vi "ColorSensor Controller.vi"(8 "error in":errorcluster) -> ()   [LabVIEW 2019]
doc: "This VI executes continuously carrying out the current operation and responding to updates or new operations. It will often contain the timing or control code that is difficult to place directly in TeleOp. This VI generally opens all sensors and motors and isolates the rest of the robot code from knowing how the operations are carried out."
uses:
  <vilib>/Rock Robotics/WPI/Framework/Completion Status.ctl
  ColorSensor Setpoints.ctl
  ColorSensor Operations.ctl
  <vilib>/Rock Robotics/SystemInterfaces/i2clib/i2c_bus.ctl
  <vilib>/Rock Robotics/WPI/ThirdParty/Phoenix-LabVIEW/Motor Controller/Controls/CTRE_Phoenix_MotorControl_ControlMode.ctl
  Framework/Robot Global Data.vi
  <vilib>/Rock Robotics/Network Tables/NT Write Boolean.vi
panel:
  in  "Interactive Values":T1
  out "Current\nCmd":string
  in  "Buttons":cluster{"Execute Cmd":bool, "Abort Cmd":bool}
  out "Command Timing":cluster{"Start Time (ms)":u32, "Iterations":i32}
  out "Status":T3
  # "Tip: It may be helpful to observe inputs and sensor values.\nYou may also want to display tuning or debugging controls."
  # "Interactive Command: You may fill in the settings for a command\nand schedule it with the Execute button. You can observe and abort\nany command while fine tuning the code for the controller."
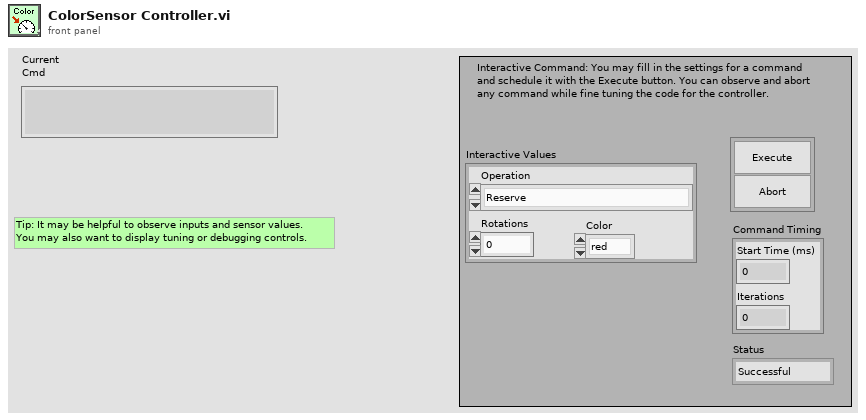
[diagram p1: front panel]
types:
  T1 = typedef "ColorSensor Setpoints.ctl" = cluster{"Operation":T2, "Rotations":dbl, "Color":enum16{"red", "blue", "yellow", "green"}}
  T2 = typedef "ColorSensor Operations.ctl" = enum16{"Reserve", "Read Current", "spin_to_color", "ColorSpin", "Immediate"}
  T3 = typedef "Completion Status.ctl" = enum16{"Successful", "Aborted", "Incomplete"}
  T4 = typedef "i2c_bus.ctl" = enum16{"I2C On-Board", "I2C MXP", "Invalid"}
  T5 = typedef "Color Sensor V3 DevRef.ctl" = cluster{"I2CDevRef":T6}
  T6 = typedef "WPI_I2CDevRef.ctl" = cluster{"DevStatus":errorcluster, "Device Address":u8, "Handle":i32, "I2C Bus":T4}
  T7 = typedef "WPI_MotorControlDeviceRef.ctl" = cluster{"DeviceStatus":errorcluster, "Type":T8, "PWM":cluster{"PWM Channel":T9, "DeadBand":T10}, "CAN":cluster{"Device Number":u8, "SetOutput VI Ref":variant, "GetOutput VI Ref":variant, "Enable VI Ref":variant, "Disable VI Ref":variant, "Data":variant}, "Invert":bool, "DIO PWM":cluster{"PWM \"Enable\" Channel":T9, "DIOChannel":T11, "PWM Rate":dbl}}
  T8 = typedef "WPI_MotorControlType.ctl" = enum16{"PWM", "CAN", "DIO PWM"}
  T9 = typedef "FPGA_DIOPWMChannel.ctl" = enum8{"PWM 0", "PWM 1", "PWM 2", "PWM 3", "PWM 4", "PWM 5", "PWM 6", "PWM 7", "PWM 8", "PWM 9", "PWM MXP 0", "PWM MXP 1", "PWM MXP 2", "PWM MXP 3", "PWM MXP 4", "PWM MXP 5", "PWM MXP 6", "PWM MXP 7", "PWM MXP 8", "PWM MXP 9", "Invalid"}
  T10 = typedef "WPI_PWMDeadband.ctl" = cluster{"Name":string, "maxPositivePwm":i32, "minPositivePwm":i32, "centerPwm":i32, "maxNegativePwm":i32, "minNegativePwm":i32, "angularRange":u16}
  T11 = typedef "FPGA_DIOChannel.ctl" = enum8{"DIO 0", "DIO 1", "DIO 2", "DIO 3", "DIO 4", "DIO 5", "DIO 6", "DIO 7", "DIO 8", "DIO 9", "DIO MXP 0", "DIO MXP 1", "DIO MXP 2", "DIO MXP 3", "DIO MXP 4", "DIO MXP 5", "DIO MXP 6", "DIO MXP 7", "DIO MXP 8", "DIO MXP 9", "DIO MXP 10", "DIO MXP 11", "DIO MXP 12", "DIO MXP 13", "DIO MXP 14", "DIO MXP 15", "SPI Port CS1", "SPI Port CS2", "SPI Port CS3", "SPI Port MISO", "SPI Port MOSI", "Invalid"}
  T12 = typedef "Command Status Info.ctl" = cluster{"Name":string, "Status":T3, "notifier out":T13}
  T13 = typedef "Completion Notifier.ctl" = refnum<notifier>
  T14 = cluster{"Current Command":T1, "Command Timing":cluster{"Start Time (ms)":u32, "Iterations":i32}, "Command Arguments":cluster{"Command Info":T12, "Description":string, "Default Command":T1, "queue out":refnum<queue>, "Subsystem Name":string}}
  T15 = typedef "CTRE_Phoenix_MotorControl_ControlMode.ctl" = u16
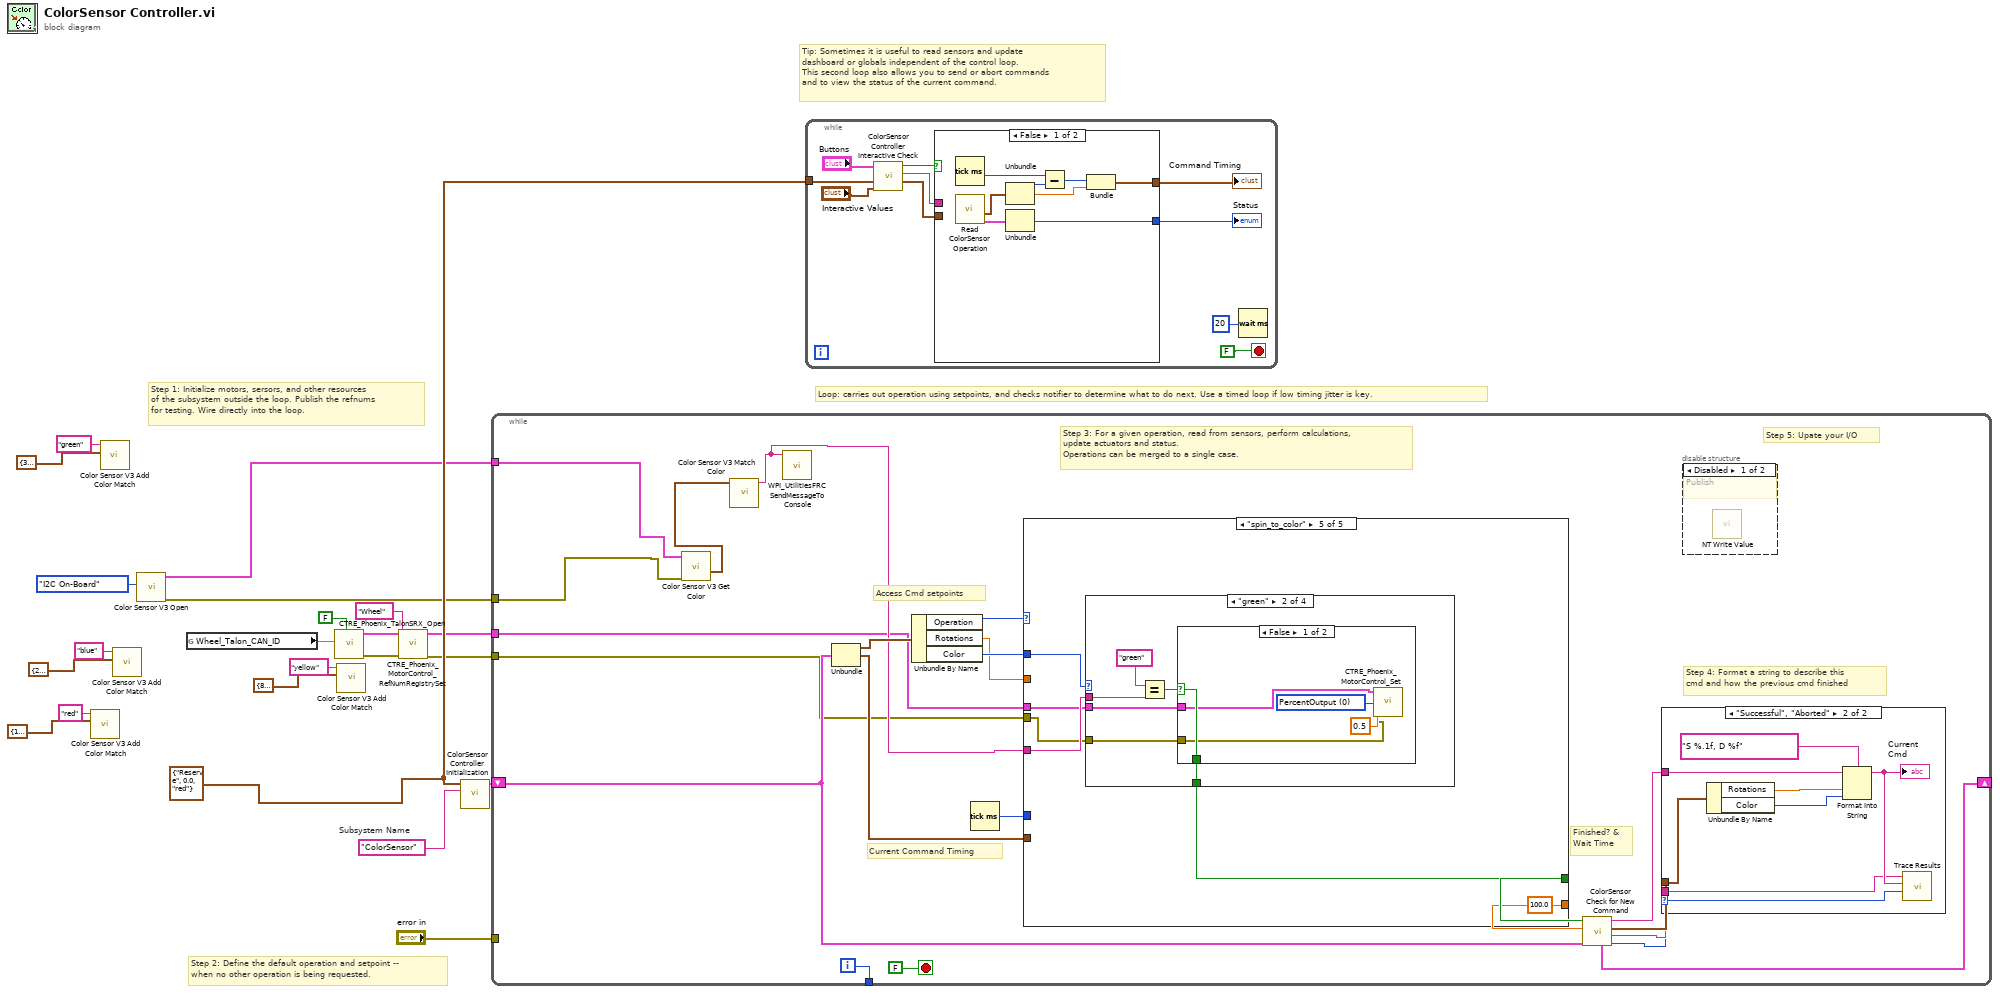
[diagram p0: block diagram]
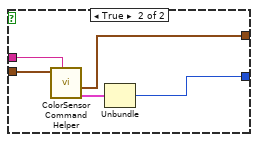
[diagram p2: hidden frame]
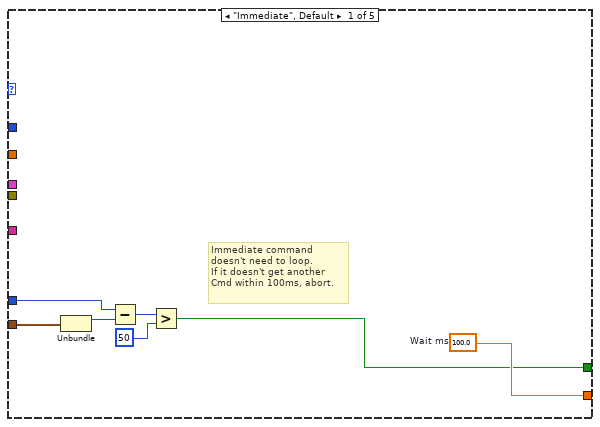
[diagram p5: hidden frame]
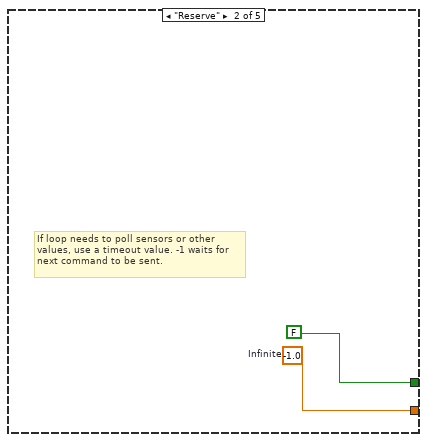
[diagram p6: hidden frame]
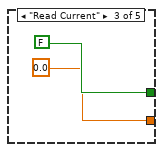
[diagram p7: hidden frame]
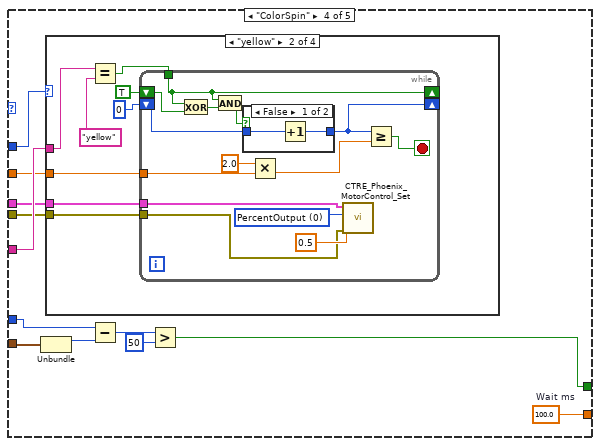
[diagram p8: hidden frame]
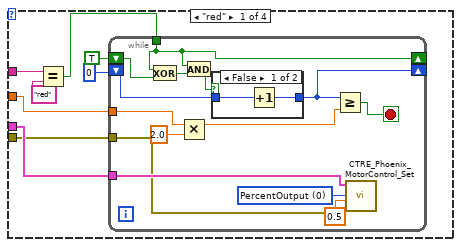
[diagram p9: hidden frame]
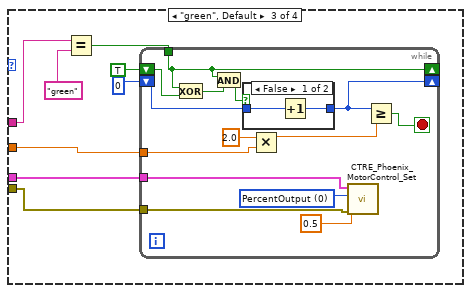
[diagram p12: hidden frame]
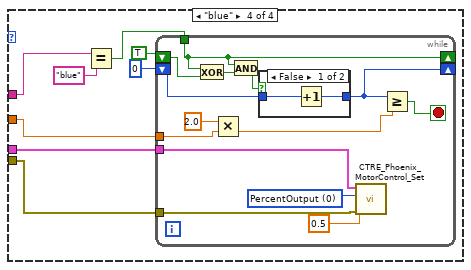
[diagram p14: hidden frame]
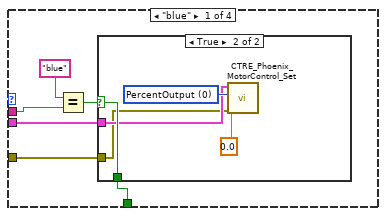
[diagram p16: hidden frame]
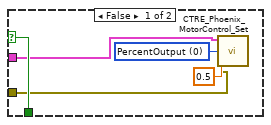
[diagram p17: hidden frame]
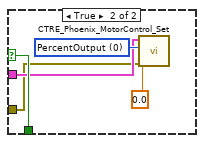
[diagram p18: hidden frame]
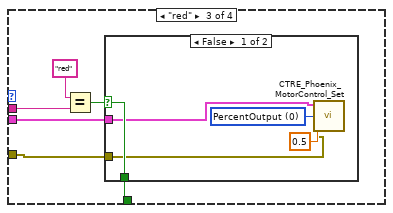
[diagram p19: hidden frame]
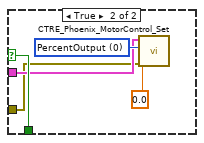
[diagram p20: hidden frame]
diagram:
  w16 = T1 {"Operation"=enum."Reserve", "Rotations"=0.0, "Color"=enum."red"} ("Default Command")
  w20 = "ColorSensor"  # Subsystem Name
  # "Tip: Sometimes it is useful to read sensors and update\ndashboard or globals independent of the control loop.\nThis second loop also allows you to send or abort commands\nand to view the status of the current command."
  # "Step 2: Define the default operation and setpoint --\nwhen no other operation is being requested."
  # "Step 1: Initialize motors, sersors, and other resources\nof the subsystem outside the loop. Publish the refnums\nfor testing. Wire directly into the loop."
  # "Loop: carries out operation using setpoints, and checks notifier to determine what to do next. Use a timed loop if low timing jitter is key."
  n1 = call <vilib>:"Color Sensor V3 Add Color Match.vi"("Color"=cluster{"R":dbl, "G":dbl, "B":dbl} {"R"=149.0, "G"=77.0, "B"=28.0}, "Name"="red") -> ()  [unwired: 10 in]
  n2 = call <vilib>:"Color Sensor V3 Add Color Match.vi"("Color"=cluster{"R":dbl, "G":dbl, "B":dbl} {"R"=39.0, "G"=149.0, "B"=66.0}, "Name"="green") -> ()  [unwired: 10 in]
  n3 = call <vilib>:"Color Sensor V3 Add Color Match.vi"("Color"=cluster{"R":dbl, "G":dbl, "B":dbl} {"R"=28.0, "G"=105.0, "B"=121.0}, "Name"="blue") -> ()  [unwired: 10 in]
  n4 = call <vilib>:"Color Sensor V3 Open.vi"("I2C Bus"=i2c_bus."I2C On-Board") -> ("error out"=w13:errorcluster, "ColorSensorDevRef"=w14:T5)  [unwired: 9 in]
  n5 = global read "Robot Global Data.vi" "Wheel_Talon_CAN_ID"() -> (w4:dbl)
  n6 = call <vilib>:"CTRE_Phoenix_TalonSRX_Open.vi"("Invert"=FALSE, "Device Number"=w4) -> ("error out"=w18:errorcluster, "CAN Talon SRX Ref"=w19:T7)  [unwired: 8 in]
  n7 = call <vilib>:"Color Sensor V3 Add Color Match.vi"("Color"=cluster{"R":dbl, "G":dbl, "B":dbl} {"R"=85.0, "G"=141.0, "B"=28.0}, "Name"="yellow") -> ()  [unwired: 10 in]
  n8 = call <vilib>:"CTRE_Phoenix_MotorControl_RefNumRegistrySet.vi"("error in (no error)"=w18, "refnum name"="Wheel", "PhoenixMotorControlDevRef"=w19) -> ("error out"=w1:errorcluster, "PhoenixMotorControlDevRef"=w2:T7)  [unwired: 7 in]
  n9 = call "ColorSensor Controller Initialization.vi"("Subsystem Name"=w20, "Default Command"=w16) -> ("Current Command"=w21:T14)  [unwired: 9 in]
  n10 = while {
    shift-right: [w38] -> _
    shift-left: w21 -> [w31]
    tunnel: [w43] -> _
    tunnel: "error in" -> [_]
    tunnel: w14 -> [w27]
    tunnel: w13 -> [w26]
    tunnel: w2 -> [w24]
    tunnel: w1 -> [w23]
    i -> [w43]
    stop <- FALSE stop-if-true
    # "Step 5: Upate your I/O"
    # "Step 4: Format a string to describe this\ncmd and how the previous cmd finished"
    # "Current Command Timing"
    # "Access Cmd setpoints"
    # "Finished? &\nWait Time"
    # "Step 3: For a given operation, read from sensors, perform calculations,\nupdate actuators and status.\nOperations can be merged to a single case."
    n11 = call <vilib>:"Color Sensor V3 Get Color.vi"("error in (no error)"=w26, "ColorSensorDevRef"=w27) -> ("Normalized Color"=w25:cluster{"R":dbl, "G":dbl, "B":dbl})  [unwired: 6 in, 3 out]
    n12 = call <vilib>:"Color Sensor V3 Match Color.vi"("Measured Color"=w25) -> ("Matched Color Name"=w28:string)  [unwired: 8 in, 2 out]
    n13 = call <vilib>:"WPI_UtilitiesFRC SendMessageToConsole.vi"("Message"=w28) -> ()  [unwired: 14 in, 1 out]
    n14 = Unbundle(w31) -> ("Current Command"=w42:T1, "Command Timing"=w39:cluster{"Start Time (ms)":u32, "Iterations":i32})  [unwired: 1 out]
    n15 = Unbundle By Name(w42) -> ("Operation"=w41:T2, "Rotations"=w29:dbl, "Color"=w30:enum16{"red", "blue", "yellow", "green"})
    n16 = Tick Count (ms)() -> (millisecond timer value=w40:u32)
    n17 = case shown="\"spin_to_color\"" w41 {
      tunnel: [w59 w61 0.0 ("Infinite") w68 100.0 ("Wait ms")] -> w36
      tunnel: [w53 FALSE ("ignore previous (F)") FALSE ("ignore previous (F)") w69 w180] -> w37
      tunnel: w39 -> [w55 _ _ w71 _]
      tunnel: w40 -> [w54 _ _ w70 _]
      tunnel: w28 -> [_ _ _ w73 w181]
      tunnel: w30 -> [_ _ _ w67 w178]
      tunnel: w29 -> [_ _ _ w66 _]
      tunnel: w24 -> [_ _ _ w65 w177]
      tunnel: w23 -> [_ _ _ w64 w176]
      frame "Immediate", Default {
        w59 = 100.0  # Wait ms
        # "Immediate command\ndoesn't need to loop.\nIf it doesn't get another\nCmd within 100ms, abort."
        n18 = Unbundle(w55) -> ("Start Time (ms)"=w58:u32)  [unwired: 1 out]
        n19 = Subtract(x=w54, y=w58) -> (x-y=w57:u32)
        n20 = Greater?(x=w57, y=u8 50 ("Left Motor")) -> (0:w53:bool)
      }
      frame "Reserve" {
        w61 = -1.0  # Infinite
        # "If loop needs to poll sensors or other\nvalues, use a timeout value. -1 waits for\nnext command to be sent."
      }
      frame "Read Current" {
      }
      frame "ColorSpin" {
        w68 = 100.0  # Wait ms
        n21 = Unbundle(w71) -> ("Start Time (ms)"=w72:u32)  [unwired: 1 out]
        n22 = case shown="\"yellow\"" w67 {
          tunnel: w73 -> [w79 w104 w129 w154]
          tunnel: w66 -> [w78 w103 w128 w153]
          tunnel: w65 -> [w77 w102 w127 w152]
          tunnel: w64 -> [w76 w101 w126 w151]
          frame "red" {
            n23 = Equal?(x=w79, y="red") -> (x = y?=w81:bool)
            n24 = while {
              shift-right: [w89] -> _
              shift-left: TRUE -> [w96]
              shift-right: [w93] -> _
              shift-left: 0 -> [w97]
              tunnel: w81 -> [w89]
              tunnel: w78 -> [w86]
              tunnel: w77 -> [w85]
              tunnel: w76 -> [w84]
              stop <- w92 stop-if-true
              w90 = T15 0 items=["PercentOutput"=0, "Position"=1, "Velocity"=2, "Current"=3, "Follower"=5, "MotionProfile"=6, "MotionMagic"=7, "MotionProfileArc"=10, "Disabled"=15] ("Control Mode")
              n25 = Exclusive Or(1:w96, 2:w89) -> (0:w95:bool)
              n26 = Multiply(x=w86, y=2.0) -> (x*y=w88:dbl)
              n27 = And(x=w89, y=w95) -> (x .and. y?=w94:bool)
              n28 = case shown="False" w94 {
                tunnel: w97 -> [w98 w100]
                tunnel: [w99 w100] -> w93
                frame False {
                  n29 = Increment(x=w98) -> (x+1=w99:i32)
                }
                frame True {
                }
              }
              n30 = Greater Or Equal?(x=w93, y=w88) -> (x >= y?=w92:bool)
              n31 = call <vilib>:"CTRE_Phoenix_MotorControl_Set.vi"("error in (no error)"=w84, "Output"=0.5, "Control Mode"=w90, "PhoenixMotorControlDevRef"=w85) -> ()  [unwired: 6 in, 2 out]
            }
          }
          frame "yellow" {
            n32 = Equal?(x=w104, y="yellow") -> (x = y?=w107:bool)
            n33 = while {
              shift-right: [w119] -> _
              shift-left: TRUE -> [w121]
              tunnel: w107 -> [w119]
              shift-right: [w117] -> _
              shift-left: 0 -> [w122]
              tunnel: w103 -> [w111]
              tunnel: w102 -> [w110]
              tunnel: w101 -> [w109]
              stop <- w116 stop-if-true
              w115 = T15 0 items=["PercentOutput"=0, "Position"=1, "Velocity"=2, "Current"=3, "Follower"=5, "MotionProfile"=6, "MotionMagic"=7, "MotionProfileArc"=10, "Disabled"=15] ("Control Mode")
              n34 = Exclusive Or(1:w121, 2:w119) -> (0:w120:bool)
              n35 = And(x=w119, y=w120) -> (x .and. y?=w118:bool)
              n36 = case shown="False" w118 {
                tunnel: w122 -> [w123 w125]
                tunnel: [w124 w125] -> w117
                frame False {
                  n37 = Increment(x=w123) -> (x+1=w124:i32)
                }
                frame True {
                }
              }
              n38 = Multiply(x=2.0, y=w111) -> (x*y=w113:dbl)
              n39 = call <vilib>:"CTRE_Phoenix_MotorControl_Set.vi"("error in (no error)"=w109, "Output"=0.5, "Control Mode"=w115, "PhoenixMotorControlDevRef"=w110) -> ()  [unwired: 6 in, 2 out]
              n40 = Greater Or Equal?(x=w117, y=w113) -> (x >= y?=w116:bool)
            }
          }
          frame "green", Default {
            n41 = Equal?(x=w129, y="green") -> (x = y?=w131:bool)
            n42 = while {
              shift-right: [w144] -> _
              shift-left: TRUE -> [w146]
              tunnel: w131 -> [w144]
              shift-right: [w142] -> _
              shift-left: 0 -> [w147]
              tunnel: w128 -> [w136]
              tunnel: w127 -> [w135]
              tunnel: w126 -> [w134]
              stop <- w141 stop-if-true
              w140 = T15 0 items=["PercentOutput"=0, "Position"=1, "Velocity"=2, "Current"=3, "Follower"=5, "MotionProfile"=6, "MotionMagic"=7, "MotionProfileArc"=10, "Disabled"=15] ("Control Mode")
              n43 = Exclusive Or(1:w146, 2:w144) -> (0:w145:bool)
              n44 = And(x=w144, y=w145) -> (x .and. y?=w143:bool)
              n45 = case shown="False" w143 {
                tunnel: w147 -> [w148 w150]
                tunnel: [w149 w150] -> w142
                frame False {
                  n46 = Increment(x=w148) -> (x+1=w149:i32)
                }
                frame True {
                }
              }
              n47 = Multiply(x=2.0, y=w136) -> (x*y=w138:dbl)
              n48 = call <vilib>:"CTRE_Phoenix_MotorControl_Set.vi"("error in (no error)"=w134, "Output"=0.5, "Control Mode"=w140, "PhoenixMotorControlDevRef"=w135) -> ()  [unwired: 6 in, 2 out]
              n49 = Greater Or Equal?(x=w142, y=w138) -> (x >= y?=w141:bool)
            }
          }
          frame "blue" {
            n50 = Equal?(x=w154, y="blue") -> (x = y?=w157:bool)
            n51 = while {
              shift-right: [w169] -> _
              shift-left: TRUE -> [w171]
              tunnel: w157 -> [w169]
              shift-right: [w167] -> _
              shift-left: 0 -> [w172]
              tunnel: w153 -> [w162]
              tunnel: w152 -> [w160]
              tunnel: w151 -> [w159]
              stop <- w166 stop-if-true
              w165 = T15 0 items=["PercentOutput"=0, "Position"=1, "Velocity"=2, "Current"=3, "Follower"=5, "MotionProfile"=6, "MotionMagic"=7, "MotionProfileArc"=10, "Disabled"=15] ("Control Mode")
              n52 = Exclusive Or(1:w171, 2:w169) -> (0:w170:bool)
              n53 = Multiply(x=2.0, y=w162) -> (x*y=w161:dbl)
              n54 = And(x=w169, y=w170) -> (x .and. y?=w168:bool)
              n55 = case shown="False" w168 {
                tunnel: w172 -> [w173 w175]
                tunnel: [w174 w175] -> w167
                frame False {
                  n56 = Increment(x=w173) -> (x+1=w174:i32)
                }
                frame True {
                }
              }
              n57 = call <vilib>:"CTRE_Phoenix_MotorControl_Set.vi"("error in (no error)"=w159, "Output"=0.5, "Control Mode"=w165, "PhoenixMotorControlDevRef"=w160) -> ()  [unwired: 6 in, 2 out]
              n58 = Greater Or Equal?(x=w167, y=w161) -> (x >= y?=w166:bool)
            }
          }
        }
        n59 = Subtract(x=w70, y=w72) -> (x-y=w75:u32)
        n60 = Greater?(x=w75, y=u8 50 ("Left Motor")) -> (0:w69:bool)
      }
      frame "spin_to_color" {
        n61 = case shown="\"green\"" w178 {
          tunnel: w181 -> [w185 w201 w217 w235]
          tunnel: [w184 w200 w216 w232] -> w180
          tunnel: w177 -> [w183 w199 w214 w231]
          tunnel: w176 -> [w182 w198 w215 w230]
          frame "blue" {
            n62 = Equal?(x="blue", y=w185) -> (x = y?=w186:bool)
            n63 = case shown="True" w186 {
              selector: w186 -> [w192 w195]
              tunnel: [w192 w195] -> w184
              tunnel: w183 -> [w189 w194]
              tunnel: w182 -> [w188 w193]
              frame False {
                w191 = T15 0 items=["PercentOutput"=0, "Position"=1, "Velocity"=2, "Current"=3, "Follower"=5, "MotionProfile"=6, "MotionMagic"=7, "MotionProfileArc"=10, "Disabled"=15] ("Control Mode")
                n64 = call <vilib>:"CTRE_Phoenix_MotorControl_Set.vi"("error in (no error)"=w188, "Output"=0.5, "Control Mode"=w191, "PhoenixMotorControlDevRef"=w189) -> ()  [unwired: 6 in, 2 out]
              }
              frame True {
                w197 = T15 0 items=["PercentOutput"=0, "Position"=1, "Velocity"=2, "Current"=3, "Follower"=5, "MotionProfile"=6, "MotionMagic"=7, "MotionProfileArc"=10, "Disabled"=15] ("Control Mode")
                n65 = call <vilib>:"CTRE_Phoenix_MotorControl_Set.vi"("error in (no error)"=w193, "Output"=0.0, "Control Mode"=w197, "PhoenixMotorControlDevRef"=w194) -> ()  [unwired: 6 in, 2 out]
              }
            }
          }
          frame "green" {
            n66 = Equal?(x="green", y=w201) -> (x = y?=w202:bool)
            n67 = case shown="False" w202 {
              selector: w202 -> [w208 w211]
              tunnel: [w208 w211] -> w200
              tunnel: w199 -> [w205 w210]
              tunnel: w198 -> [w204 w209]
              frame False {
                w207 = T15 0 items=["PercentOutput"=0, "Position"=1, "Velocity"=2, "Current"=3, "Follower"=5, "MotionProfile"=6, "MotionMagic"=7, "MotionProfileArc"=10, "Disabled"=15] ("Control Mode")
                n68 = call <vilib>:"CTRE_Phoenix_MotorControl_Set.vi"("error in (no error)"=w204, "Output"=0.5, "Control Mode"=w207, "PhoenixMotorControlDevRef"=w205) -> ()  [unwired: 6 in, 2 out]
              }
              frame True {
                w213 = T15 0 items=["PercentOutput"=0, "Position"=1, "Velocity"=2, "Current"=3, "Follower"=5, "MotionProfile"=6, "MotionMagic"=7, "MotionProfileArc"=10, "Disabled"=15] ("Control Mode")
                n69 = call <vilib>:"CTRE_Phoenix_MotorControl_Set.vi"("error in (no error)"=w209, "Output"=0.0, "Control Mode"=w213, "PhoenixMotorControlDevRef"=w210) -> ()  [unwired: 6 in, 2 out]
              }
            }
          }
          frame "red" {
            n70 = Equal?(x="red", y=w217) -> (x = y?=w218:bool)
            n71 = case shown="False" w218 {
              selector: w218 -> [w224 w227]
              tunnel: [w224 w227] -> w216
              tunnel: w215 -> [w221 w225]
              tunnel: w214 -> [w220 w226]
              frame False {
                w223 = T15 0 items=["PercentOutput"=0, "Position"=1, "Velocity"=2, "Current"=3, "Follower"=5, "MotionProfile"=6, "MotionMagic"=7, "MotionProfileArc"=10, "Disabled"=15] ("Control Mode")
                n72 = call <vilib>:"CTRE_Phoenix_MotorControl_Set.vi"("error in (no error)"=w221, "Output"=0.5, "Control Mode"=w223, "PhoenixMotorControlDevRef"=w220) -> ()  [unwired: 6 in, 2 out]
              }
              frame True {
                w229 = T15 0 items=["PercentOutput"=0, "Position"=1, "Velocity"=2, "Current"=3, "Follower"=5, "MotionProfile"=6, "MotionMagic"=7, "MotionProfileArc"=10, "Disabled"=15] ("Control Mode")
                n73 = call <vilib>:"CTRE_Phoenix_MotorControl_Set.vi"("error in (no error)"=w225, "Output"=0.0, "Control Mode"=w229, "PhoenixMotorControlDevRef"=w226) -> ()  [unwired: 6 in, 2 out]
              }
            }
          }
          frame "yellow" {
            n74 = Equal?(x="yellow", y=w235) -> (x = y?=w233:bool)
            n75 = case shown="False" w233 {
              selector: w233 -> [w240 w243]
              tunnel: [w240 w243] -> w232
              tunnel: w231 -> [w237 w242]
              tunnel: w230 -> [w236 w241]
              frame False {
                w239 = T15 0 items=["PercentOutput"=0, "Position"=1, "Velocity"=2, "Current"=3, "Follower"=5, "MotionProfile"=6, "MotionMagic"=7, "MotionProfileArc"=10, "Disabled"=15] ("Control Mode")
                n76 = call <vilib>:"CTRE_Phoenix_MotorControl_Set.vi"("error in (no error)"=w236, "Output"=0.5, "Control Mode"=w239, "PhoenixMotorControlDevRef"=w237) -> ()  [unwired: 6 in, 2 out]
              }
              frame True {
                w245 = T15 0 items=["PercentOutput"=0, "Position"=1, "Velocity"=2, "Current"=3, "Follower"=5, "MotionProfile"=6, "MotionMagic"=7, "MotionProfileArc"=10, "Disabled"=15] ("Control Mode")
                n77 = call <vilib>:"CTRE_Phoenix_MotorControl_Set.vi"("error in (no error)"=w241, "Output"=0.0, "Control Mode"=w245, "PhoenixMotorControlDevRef"=w242) -> ()  [unwired: 6 in, 2 out]
              }
            }
          }
        }
      }
    }
    n78 = call "ColorSensor Check for New Command.vi"("Current Command"=w31, "Wait time (ms)"=w36, "Finished?"=w37) -> ("Completion"=w32:T3, "Subsystem Name"=w33:string, "Current Command"=w34:T1, "Initial Trace String"=w35:string, "NextCommand"=w38:T14)  [unwired: 4 in]
    n79 = case shown="\"Successful\", \"Aborted\"" w32 {
      selector: w32 -> [_ w52]
      tunnel: w35 -> [_ w48]
      tunnel: w34 -> [_ w49]
      tunnel: w33 -> [_ w45]
      frame "Incomplete", Default {
        # "Continuing current command"
      }
      frame "Successful", "Aborted" {
        # "Report and setup for next command"
        n80 = Unbundle By Name(w49) -> ("Rotations"=w51:dbl, "Color"=w46:enum16{"red", "blue", "yellow", "green"})
        n81 = Format Into String(format string="S %.1f, D %f", initial string=w48, w51, w46) -> (resulting string=w47:string)  [unwired: 1 in, 1 out]
        "Current\nCmd" <- w47
        n82 = call <vilib>:"Trace Results.vi"("Status of previous command"=w52, "Description"=w47, "Subsystem"=w45) -> ()  [unwired: 9 in]
      }
    }
    n83 = disable-structure shown="Disabled" {
      frame Disabled {
        # "Publish"
        n84 = call-poly <vilib>:"NT Write Value.vi"() -> ()  [unwired: 11 in, 1 out]
      }
      frame Enabled {
      }
    }
  }
  n85 = while {
    tunnel: w16 -> [w252]
    stop <- FALSE stop-if-true
    n86 = call "ColorSensor Controller Interactive Check.vi"("Interactive Command in"="Interactive Values", "Default Command"=w252, "Buttons"="Buttons") -> ("Interactive Command out"=w249:T1, "Trace String"=w250:string, "Schedule"=w251:bool)  [unwired: 6 in]
    n87 = case shown="False" w251 {
      tunnel: [w263 w268] -> w248
      tunnel: w249 -> [_ w266]
      tunnel: [w259 w264] -> w247
      tunnel: w250 -> [_ w267]
      frame False {
        n88 = Tick Count (ms)() -> (millisecond timer value=w258:u32)
        n89 = call "Read ColorSensor Operation.vi"() -> ("Command Info"=w256:T12, "SubSystem Data"=w257:T1)  [unwired: 9 in, 1 out]
        n90 = Unbundle(w257) -> ("Operation"=w262:T2, "Rotations"=w260:dbl)  [unwired: 1 out]
        n91 = Unbundle(w256) -> ("Status"=w263:T3)  [unwired: 2 out]
        n92 = Subtract(x=w258, y=w262) -> (x-y=w261:u32)
        n93 = Bundle(w261, "Rotations"=w260) -> (w259:cluster{u32, "Rotations":dbl})  [unwired: 1 in]
      }
      frame True {
        n94 = call "ColorSensor Command Helper.vi"("Description"=w267, "SubSystem Data"=w266) -> ("Command Info Out"=w265:T12, "Command Timing"=w264:cluster{"Start Time (ms)":u32, "Iterations":i32})  [unwired: 7 in, 1 out]
        n95 = Unbundle(w265) -> ("Status"=w268:T3)  [unwired: 2 out]
      }
    }
    "Status" <- w248
    "Command Timing" <- w247
    n96 = Wait (ms)(milliseconds to wait=u32 20) -> ()  [unwired: 1 out]
  }
